vi "fileIO.vi"() -> ()   [LabVIEW 2014]
panel:
  in  "stop":bool
  out "concatenated string":string
  in  "Frequency (Hz)":u32
  in  "File Name":string
  in  "file path (use dialog)":path
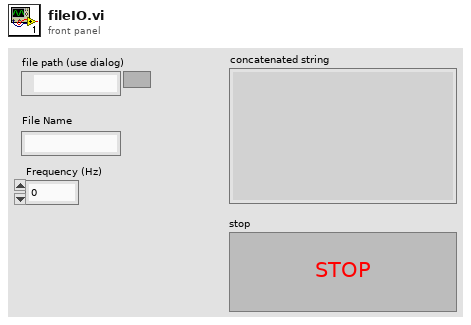
[diagram p1: front panel]
types:
  T1 = enum16{"open", "replace", "create", "open or create", "replace or create", "replace or create with confirmation"}
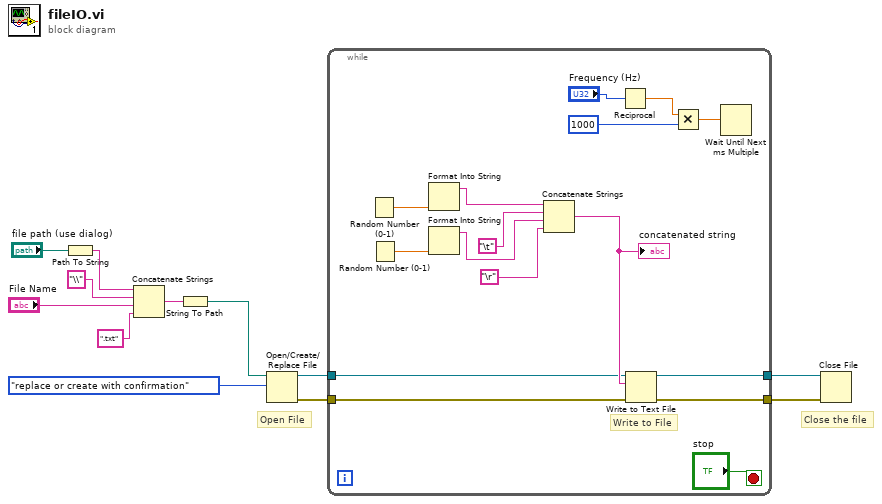
[diagram p0: block diagram]
diagram:
  # "Close the file"
  # "Open File"
  n1 = Path To String(path="file path (use dialog)") -> (string=w6:string)
  n2 = Concatenate Strings(w6, "\\" ("string"), "File Name", ".txt" ("string")) -> (w2:string)
  n3 = String To Path(string=w2) -> (path=w1:path)
  n4 = Open/Create/Replace File(file path (use dialog)=w1, operation (0:open)=T1."replace or create with confirmation") -> (refnum out=w12:refnum<file>, error out=w11:errorcluster)  [unwired: 4 in, 1 out]
  n5 = while {
    tunnel: w12 -> [w21]
    tunnel: w11 -> [w20]
    tunnel: [w19] -> w10
    tunnel: [w18] -> w9
    stop <- "stop" stop-if-true
    # "Write to File"
    n6 = Random Number (0-1)() -> (number: 0 to 1=w28:dbl)
    n7 = Random Number (0-1)() -> (number: 0 to 1=w27:dbl)
    n8 = Format Into String(w28) -> (resulting string=w26:string)  [unwired: 3 in, 1 out]
    n9 = Format Into String(w27) -> (resulting string=w24:string)  [unwired: 3 in, 1 out]
    n10 = Concatenate Strings(w26, "\t", w24, "\r") -> (w22:string)
    "concatenated string" <- w22
    n11 = Reciprocal(x="Frequency (Hz)") -> (1/x=w13:dbl)
    n12 = Write to Text File(file (use dialog)=w21, text=w22, error in=w20) -> (refnum out=w19:refnum<file>, error out=w18:errorcluster)  [unwired: 1 in, 1 out]
    n13 = Multiply(x=w13, y=u32 1000) -> (x*y=w15:dbl)
    n14 = Wait Until Next ms Multiple(millisecond multiple=w15) -> ()  [unwired: 1 out]
  }
  n15 = Close File(refnum=w10, error in=w9) -> ()  [unwired: 2 out]
